vi "Generador de Funciones Arbitrarias v0.1.vi"() -> ()   [LabVIEW 2016]
panel:
  in  "Muestras":i32(knob) scale=100.0..2000.0
  in  "Ciclo de Trabajo":i32(knob) scale=0.0..100.0
  in  "Desfase":dbl(knob) scale=-180.0..180.0
  in  "Offseet":dbl(slide) scale=-50.0..100.0
  in  "Frecuencia":dbl(slide) scale=0.0..10.0
  in  "Amplitud":dbl(slide) scale=0.0..100.0
  out "Waveform Graph":dbl[](graph)
  in  "Estado Anterior":bool
  in  "Estado Siguiente":bool
  out "Constante":bool
  out "PWM":bool
  out "Sinusoidal":bool
  out "Ruido":bool
  out "Rampa":bool
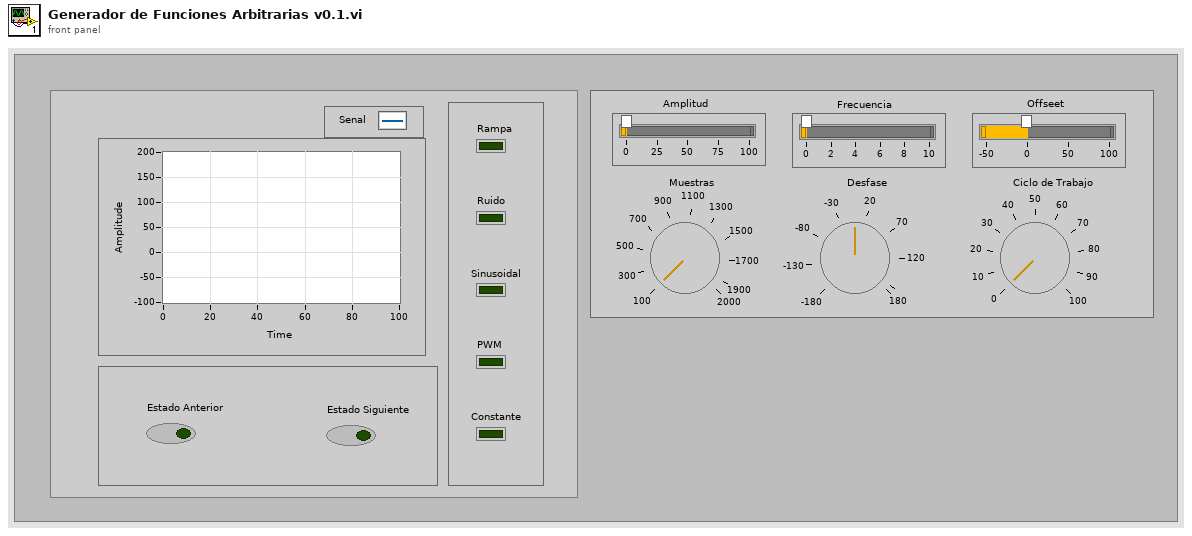
[diagram p1: front panel]
types:
  T1 = enum16{"State_1", "State_2", "State_3", "State_4", "State_5"}
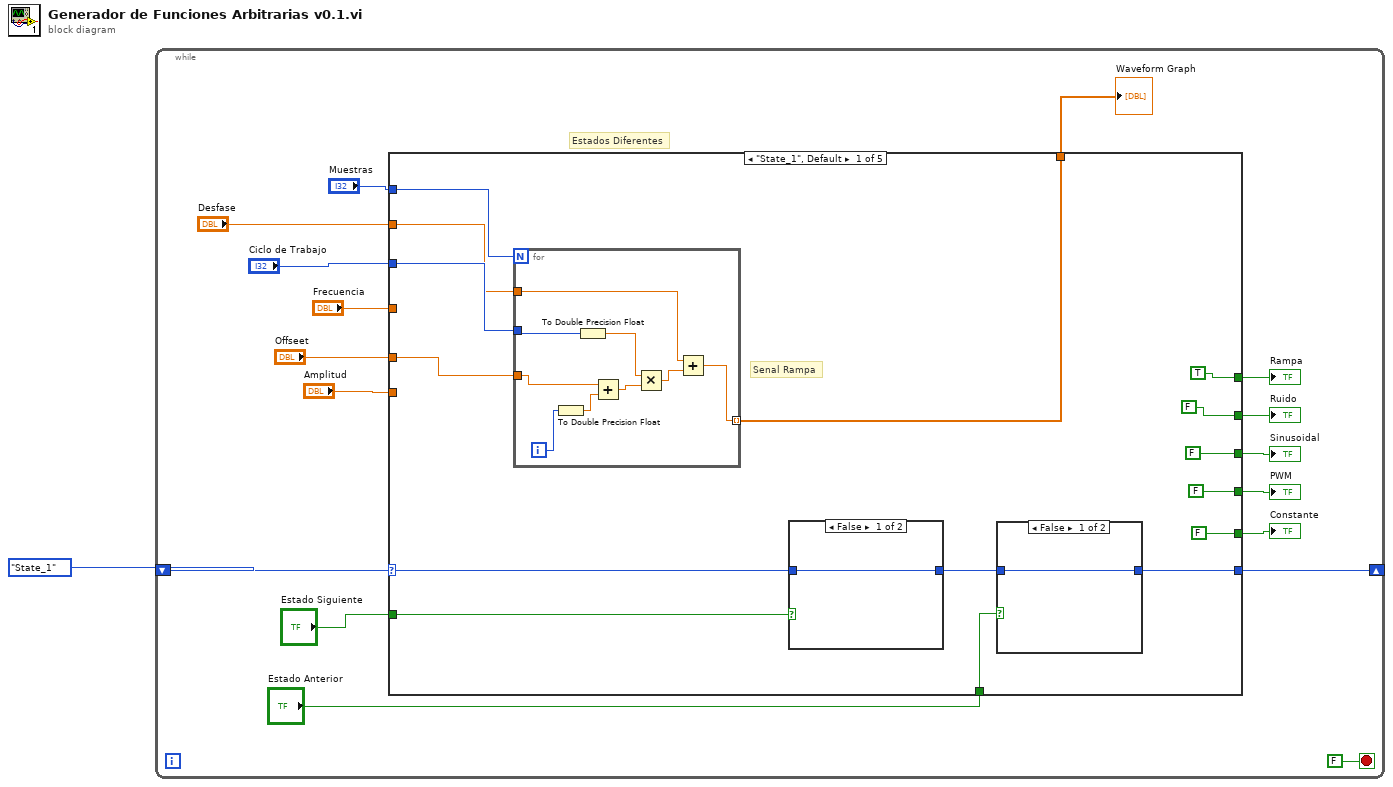
[diagram p0: block diagram]
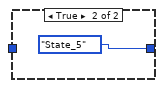
[diagram p2: hidden frame]
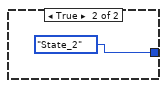
[diagram p3: hidden frame]
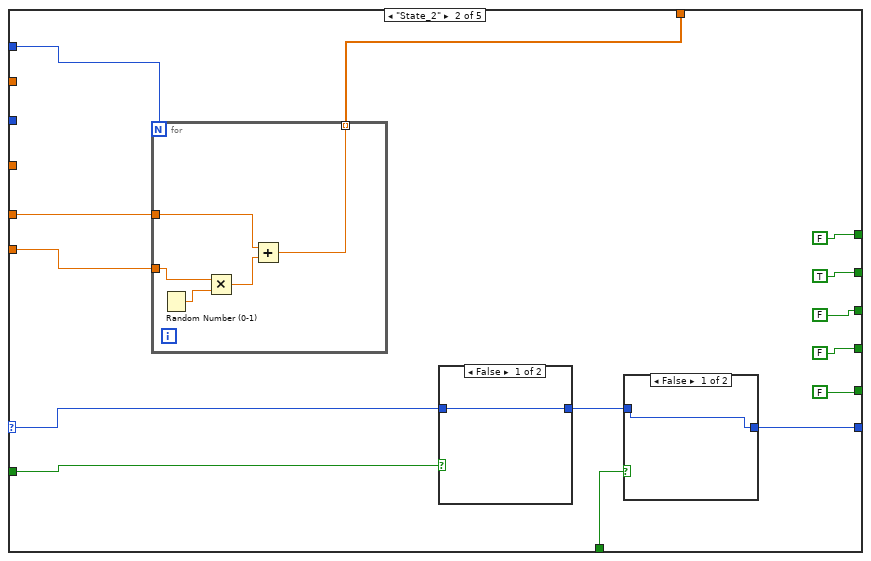
[diagram p4: hidden frame]
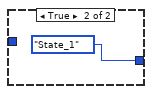
[diagram p5: hidden frame]
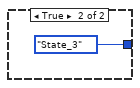
[diagram p6: hidden frame]
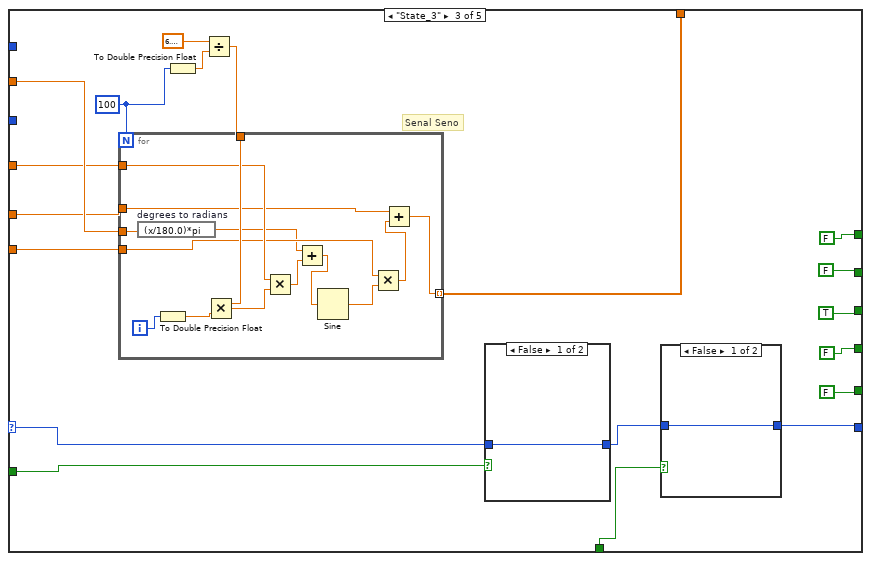
[diagram p7: hidden frame]
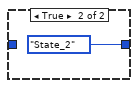
[diagram p8: hidden frame]
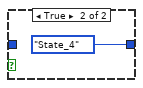
[diagram p9: hidden frame]
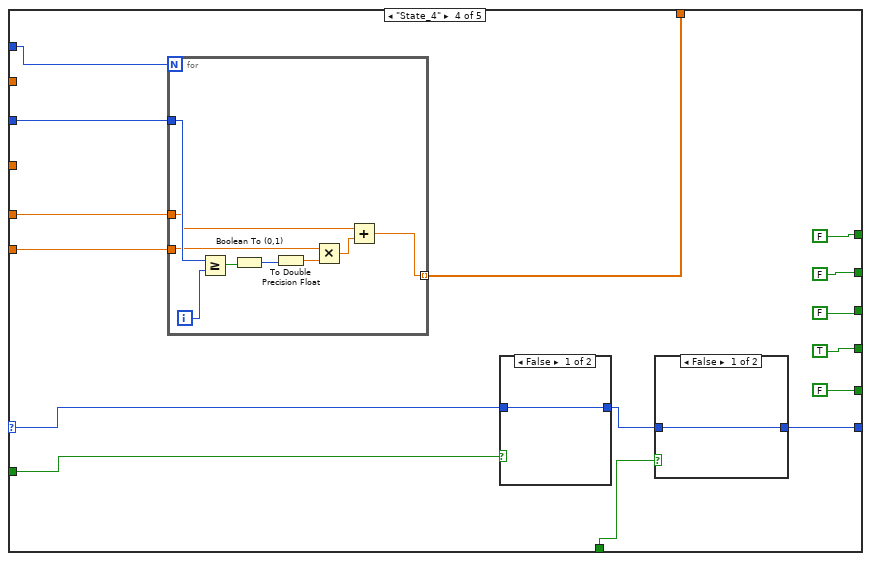
[diagram p10: hidden frame]
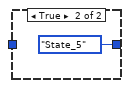
[diagram p11: hidden frame]
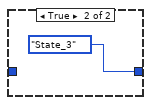
[diagram p12: hidden frame]
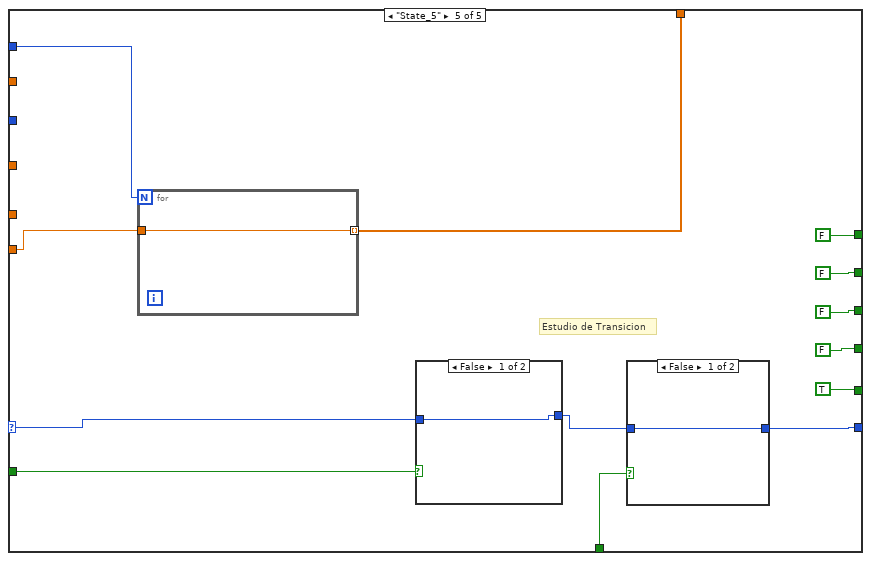
[diagram p13: hidden frame]
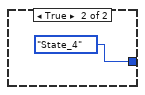
[diagram p14: hidden frame]
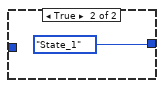
[diagram p15: hidden frame]
diagram:
  n1 = while {
    shift-right: [w17] -> _
    shift-left: T1."State_1" -> [w18]
    stop <- FALSE stop-if-true
    # "Estados Diferentes"
    n2 = case shown="\"State_1\", Default" w18 {
      selector: w18 -> [w26 w53 w81 w114 w140]
      tunnel: [w25 w52 w80 w113 w138] -> w17
      tunnel: [FALSE TRUE FALSE FALSE FALSE] -> w16
      tunnel: [TRUE FALSE FALSE FALSE FALSE] -> w15
      tunnel: [FALSE FALSE TRUE FALSE FALSE] -> w14
      tunnel: [FALSE FALSE FALSE TRUE FALSE] -> w13
      tunnel: [FALSE FALSE FALSE FALSE TRUE] -> w12
      tunnel: "Estado Siguiente" -> [w27 w54 w83 w115 w141]
      tunnel: "Estado Anterior" -> [w28 w55 w82 w116 w142]
      tunnel: [w23 w50 w74 w111 w137] -> w8
      tunnel: "Ciclo de Trabajo" -> [w22 _ _ w109 _]
      tunnel: "Muestras" -> [w21 w49 _ w110 w135]
      tunnel: "Desfase" -> [w20 _ w73 _ _]
      tunnel: "Amplitud" -> [_ w48 w70 w108 w136]
      tunnel: "Offseet" -> [w19 w47 w71 w107 _]
      tunnel: "Frecuencia" -> [_ _ w72 _ _]
      frame "State_1", Default {
        # "Senal Rampa"
        n3 = for {
          N: w21 -> [_]
          tunnel: [w36] -> w23 mode=indexing
          tunnel: w19 -> [w40]
          tunnel: w22 -> [w34]
          tunnel: w20 -> [w37]
          i -> [w42]
          n4 = To Double Precision Float(number=w42) -> (double precision float=w41:dbl)
          n5 = To Double Precision Float(number=w34) -> (double precision float=w35:dbl)
          n6 = Add(x=w40, y=w41) -> (x+y=w39:dbl)
          n7 = Multiply(x=w35, y=w39) -> (x*y=w38:dbl)
          n8 = Add(x=w37, y=w38) -> (x+y=w36:dbl)
        }
        n9 = case shown="False" w27 {
          tunnel: [w45 T1."State_2"] -> w24
          tunnel: w26 -> [w45 _]
          frame False {
          }
          frame True {
          }
        }
        n10 = case shown="False" w28 {
          tunnel: [w43 T1."State_5"] -> w25
          tunnel: w24 -> [w43 _]
          frame False {
          }
          frame True {
          }
        }
      }
      frame "State_2" {
        n11 = for {
          N: w49 -> [_]
          tunnel: [w61] -> w50 mode=indexing
          tunnel: w48 -> [w64]
          tunnel: w47 -> [w62]
          n12 = Random Number (0-1)() -> (number: 0 to 1=w65:dbl)
          n13 = Multiply(x=w64, y=w65) -> (x*y=w63:dbl)
          n14 = Add(x=w62, y=w63) -> (x+y=w61:dbl)
        }
        n15 = case shown="False" w54 {
          tunnel: [w68 T1."State_3"] -> w51
          tunnel: w53 -> [w68 _]
          frame False {
          }
          frame True {
          }
        }
        n16 = case shown="False" w55 {
          tunnel: [w66 T1."State_1"] -> w52
          tunnel: w51 -> [w66 _]
          frame False {
          }
          frame True {
          }
        }
      }
      frame "State_3" {
        w76 = 100
        # "Senal Seno"
        n17 = To Double Precision Float(number=w76) -> (double precision float=w77:dbl)
        n18 = Divide(x=6.283185307179586, y=w77) -> (x/y=w75:dbl)
        n19 = for {
          N: w76 -> [_]
          tunnel: w75 -> [w100]
          tunnel: [w96] -> w74 mode=indexing
          tunnel: w73 -> [w90]
          tunnel: w72 -> [w99]
          tunnel: w71 -> [w94]
          tunnel: w70 -> [w92]
          i -> [w101]
          n20 = expression code="(x/180.0)*pi" "degrees to radians"(w90) -> (w89:dbl)
          n21 = To Double Precision Float(number=w101) -> (double precision float=w102:dbl)
          n22 = Multiply(x=w100, y=w102) -> (x*y=w98:dbl)
          n23 = Multiply(x=w99, y=w98) -> (x*y=w97:dbl)
          n24 = Add(x=w89, y=w97) -> (x+y=w95:dbl)
          n25 = Sine(x=w95) -> (sin(x)=w93:dbl)
          n26 = Multiply(x=w92, y=w93) -> (x*y=w91:dbl)
          n27 = Add(x=w94, y=w91) -> (x+y=w96:dbl)
        }
        n28 = case shown="False" w83 {
          tunnel: [w105 T1."State_4"] -> w79
          tunnel: w81 -> [w105 _]
          frame False {
          }
          frame True {
          }
        }
        n29 = case shown="False" w82 {
          tunnel: [w103 T1."State_2"] -> w80
          tunnel: w79 -> [w103 _]
          frame False {
          }
          frame True {
          }
        }
      }
      frame "State_4" {
        n30 = for {
          N: w110 -> [_]
          tunnel: [w122] -> w111 mode=indexing
          tunnel: w109 -> [w128]
          tunnel: w108 -> [w125]
          tunnel: w107 -> [w123]
          i -> [w130]
          n31 = Greater Or Equal?(x=w128, y=w130) -> (x >= y?=w129:bool)
          n32 = Boolean To (0,1)(Boolean=w129) -> (0, 1=w127:i16)
          n33 = To Double Precision Float(number=w127) -> (double precision float=w126:dbl)
          n34 = Multiply(x=w125, y=w126) -> (x*y=w124:dbl)
          n35 = Add(x=w123, y=w124) -> (x+y=w122:dbl)
        }
        n36 = case shown="False" w115 {
          tunnel: [w131 T1."State_5"] -> w112
          tunnel: w114 -> [w131 _]
          frame False {
          }
          frame True {
          }
        }
        n37 = case shown="False" w116 {
          tunnel: [w133 T1."State_3"] -> w113
          tunnel: w112 -> [w133 _]
          frame False {
          }
          frame True {
          }
        }
      }
      frame "State_5" {
        # "Estudio de Transicion"
        n38 = for {
          N: w135 -> [_]
          tunnel: [w148] -> w137 mode=indexing
          tunnel: w136 -> [w148]
        }
        n39 = case shown="False" w141 {
          tunnel: [w151 T1."State_1"] -> w139
          tunnel: w140 -> [w151 _]
          frame False {
          }
          frame True {
          }
        }
        n40 = case shown="False" w142 {
          tunnel: [w149 T1."State_4"] -> w138
          tunnel: w139 -> [w149 _]
          frame False {
          }
          frame True {
          }
        }
      }
    }
    "Rampa" <- w15
    "Ruido" <- w16
    "Sinusoidal" <- w14
    "PWM" <- w13
    "Constante" <- w12
    "Waveform Graph" <- w8
  }
